vi "CW Pulse Sequence Generator.vi"(0 "Pulse Laser":bool, 1 "Pulse MW":bool, 2 "Rate (Hz)":dbl) -> (7 "Pulse Sequence Out":T1(array[cluster]))   [LabVIEW 2012]
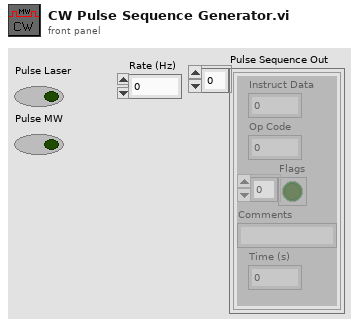
[diagram p1: front panel]
types:
  T1 = cluster{"Instruct Data":i32, "Op Code":i32, "Flags":bool[], "Comments":string, "Time (s)":dbl}[]
  T2 = cluster{"Instruct Data":i32, "Op Code":i32, "Flags":bool[], "Comments":string, "Time (s)":dbl}
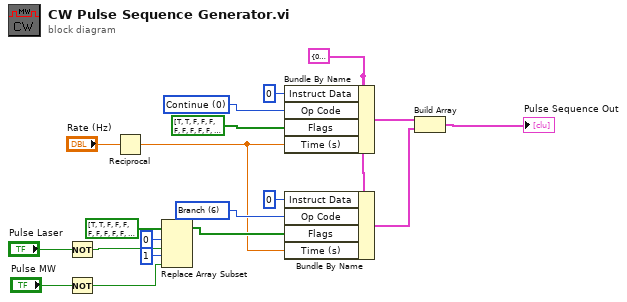
[diagram p0: block diagram]
diagram:
  w14 = 6 items=["Continue", "Stop", "Loop", "End Loop", "JSR", "RTS", "Branch", "Long Delay", "Wait"] ("Op Code")
  w13 = T2 {"Instruct Data"=0, "Op Code"=0, "Flags"=[FALSE, FALSE, FALSE, FALSE, FALSE, FALSE, FALSE, FALSE, FALSE, FALSE, FALSE, FALSE, FALSE, FALSE, FALSE, FALSE, FALSE, FALSE, FALSE, FALSE, FALSE, TRUE, TRUE, TRUE], "Comments"="", "Time (s)"=0.01} ("PB Inst 2")
  w18 = 0 items=["Continue", "Stop", "Loop", "End Loop", "JSR", "RTS", "Branch", "Long Delay", "Wait"] ("Op Code")
  n1 = Not(x="Pulse Laser") -> (.not. x?=w9:bool)
  n2 = Not(x="Pulse MW") -> (.not. x?=w6:bool)
  n3 = Reciprocal(x="Rate (Hz)") -> (1/x=w4:dbl)
  n4 = Replace Array Subset(array=bool[] [TRUE, TRUE, FALSE, FALSE, FALSE, FALSE, FALSE, FALSE, FALSE, FALSE, FALSE, FALSE, FALSE, FALSE, FALSE, FALSE, FALSE, FALSE, FALSE, FALSE, FALSE, TRUE, TRUE, TRUE] ("Flags"), new element #1=w9, index #1=0 ("index"), new element #2=w6, index #2=1 ("index")) -> (w5:bool[])
  n5 = Bundle By Name(cluster=w13, "Instruct Data"=0, "Op Code"=w18, "Flags"=bool[] [TRUE, TRUE, FALSE, FALSE, FALSE, FALSE, FALSE, FALSE, FALSE, FALSE, FALSE, FALSE, FALSE, FALSE, FALSE, FALSE, FALSE, FALSE, FALSE, FALSE, FALSE, TRUE, TRUE, TRUE], "Time (s)"=w4) -> (w3:T2)
  n6 = Bundle By Name(cluster=w13, "Instruct Data"=0, "Op Code"=w14, "Flags"=w5, "Time (s)"=w4) -> (w2:T2)
  n7 = Build Array(w3, w2) -> (→"Pulse Sequence Out":T1)
